vi "AssetInterface_Update Tags.vi"(8 "error in (no error)":errorcluster, 10 "TagBus DVR":refnum<data-value>, 11 "Asset_Interface in":refnum<class "Grid.lvclass">) -> (0 "error out":errorcluster, 2 "TagBus DVR out":refnum<data-value>, 3 "Asset_Interface out":refnum<class "Grid.lvclass">)   [LabVIEW 2015, in "Grid.lvclass"]
uses:
  Grid.lvclass
  TagBus/TagBus.lvclass
  Grid.lvclass/Grid.ctl
panel:
  out "Status":cluster{"kW":dbl}
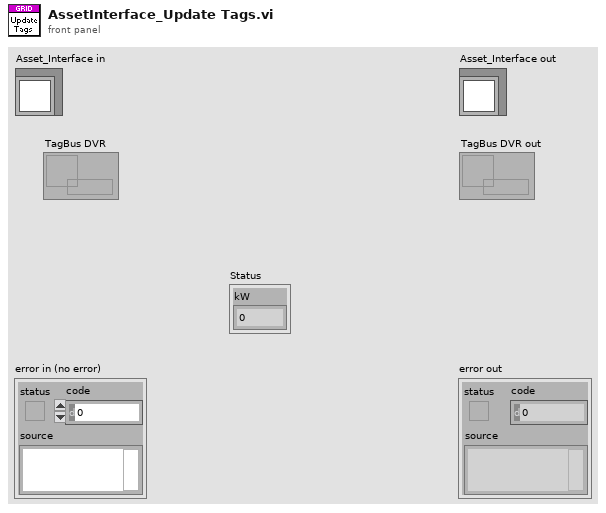
[diagram p1: front panel]
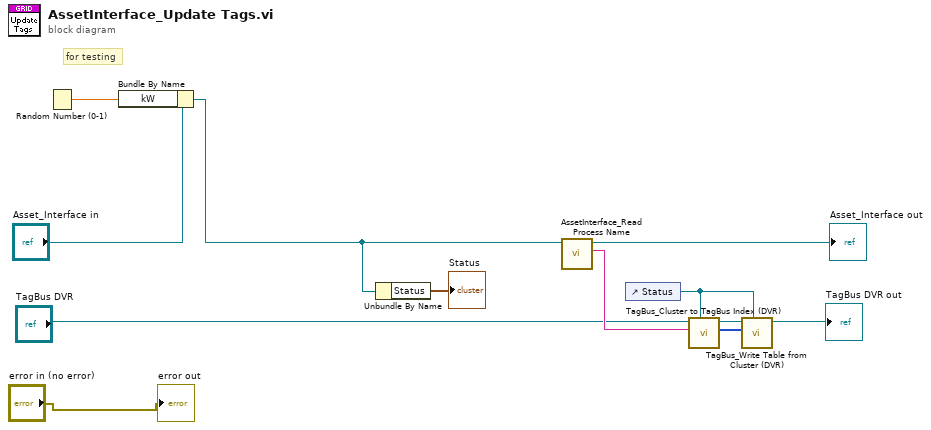
[diagram p0: block diagram]
diagram:
  # "for testing"
  n1 = Random Number (0-1)() -> (number: 0 to 1=w9:dbl)
  n2 = Bundle By Name(cluster="Asset_Interface in", "kW"=w9) -> (w10:refnum<class "Grid.lvclass">)
  n3 = Unbundle By Name(w10) -> ("Status"=→"Status":cluster{"kW":dbl})
  n4 = call-dynamic "AssetInterface_Read Process Name.vi"("Grid in"=w10) -> ("Process Name"=w5:string, "Grid out"=→"Asset_Interface out":refnum<class "Grid.lvclass">)  [unwired: 9 in]
  n5 = control-ref of="Status"() -> (w6:refnum<vi>)
  n6 = call "TagBus_Cluster to TagBus Index (DVR).vi"("Clust Refnum"=w6, "Tag Name Prepend"=w5, "TagBus DVR"="TagBus DVR") -> ("Index Array"=w7:i32[], "TagBus DVR out"=w8:refnum<data-value>)  [unwired: 7 in]
  n7 = call "TagBus_Write Table from Cluster (DVR).vi"("Clust Refnum"=w6, "Index Array"=w7, "Data Value Reference in"=w8) -> ("Data Value Reference out"=→"TagBus DVR out":refnum<data-value>)  [unwired: 8 in]
  "error out" <- "error in (no error)"
